vi "MB Serial Modbus Data Unit to String.vi"(10 "Modbus Data Unit":T2={"Function Code"=1, "Data"=[]} {"Function Code" items=["Read Coils"=1, "Read Discrete Inputs"=2, "Read Holding Registers"=3, "Read Input Registers"=4, "Write Single Coil"=5, "Write Single Register"=6, "Read Exception Status"=7, "Write Multiple Coils"=15, "Write Multiple Registers"=16]; "Data" format="%.0x"}, 11 "Serial Parameters":T1 {"Slave Address" format="%.0x"}) -> (3 "String":string)   [LabVIEW 2017]
uses:
  MB Modbus Data Unit.ctl
panel:
  # "VI Name: MB Serial Modbus Data Unit to String.vi\nPurpose: Formats the Modbus message to send.\nReentrant."
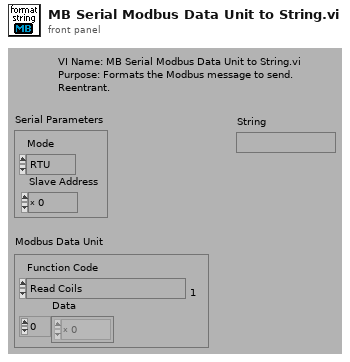
[diagram p1: front panel]
types:
  T1 = cluster{"Mode":enum16{"RTU", "ASCII"}, "Slave Address":u8}
  T2 = typedef "MB Modbus Data Unit.ctl" = cluster{"Function Code":u8, "Data":u8[]}
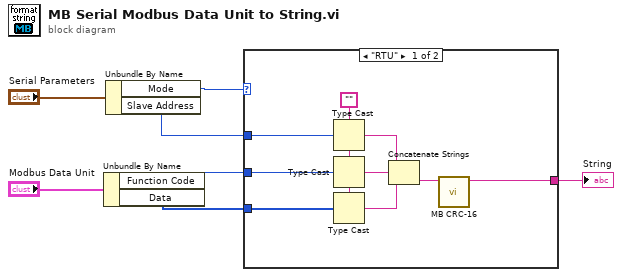
[diagram p0: block diagram]
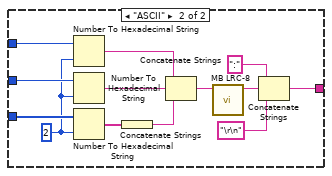
[diagram p2: hidden frame]
diagram:
  n1 = Unbundle By Name("Modbus Data Unit") -> ("Function Code"=w5:u8, "Data"=w4:u8[])
  n2 = Unbundle By Name("Serial Parameters") -> ("Mode"=w2:enum16{"RTU", "ASCII"}, "Slave Address"=w1:u8)
  n3 = case shown="\"RTU\"" w2 {
    tunnel: w1 -> [w13 w29]
    tunnel: w5 -> [w14 w28]
    tunnel: w4 -> [w15 w27]
    tunnel: [w8 w20] -> w7
    frame "RTU" {
      w16 = ""
      n4 = Type Cast(type=w16, x=w13) -> (*(type *) &x=w12:string)
      n5 = Type Cast(type=w16, x=w14) -> (*(type *) &x=w11:string)
      n6 = Type Cast(type=w16, x=w15) -> (*(type *) &x=w10:string)
      n7 = Concatenate Strings(w12, w11, w10) -> (w9:string)
      n8 = call "MB CRC-16.vi"("String"=w9) -> ("String & CRC-16"=w8:string)  [unwired: 10 out]
    }
    frame "ASCII" {
      w19 = 2
      n9 = Number To Hexadecimal String(1:w19, 2:w29) -> (0:w26:string)
      n10 = Number To Hexadecimal String(1:w19, 2:w28) -> (0:w25:string)
      n11 = Number To Hexadecimal String(1:w19, 2:w27) -> (0:w18:string[])
      n12 = Concatenate Strings(w18) -> (w17:string)
      n13 = Concatenate Strings(w26, w25, w17) -> (w24:string)
      n14 = call "MB LRC-8.vi"("String"=w24) -> ("string & LRC-8"=w22:string)  [unwired: 10 out]
      n15 = Concatenate Strings(":", w22, "\r\n") -> (w20:string)
    }
  }
  "String" <- w7
